vi "Measure Statistics (Multiple).vi"(6 "Measurements":T2[](array[typedef]), 8 "error in (no error)":errorcluster, 9 "No. Reads":i32, 10 "Channel":T3, 11 "MSOX6004 in":refnum<class "MSOX6004.lvclass">) -> (0 "error out":errorcluster, 2 "Multiple Statistics":T1(array[cluster]), 3 "MSOX6004 out":refnum<class "MSOX6004.lvclass">)   [LabVIEW 2018, in "MSOX6004.lvlib" / "MSOX6004.lvclass"]
uses:
  MSOX6004.lvclass
  PPLs/Oscilloscope/Parent/Oscilloscope.lvlibp/Custom Controls/Analog Channels.ctl
  PPLs/Oscilloscope/Parent/Oscilloscope.lvlibp/Custom Controls/Measurement.ctl
  MSOX6004.lvclass/MSOX6004.ctl
  <instrlib>/Keysight InfiniiVision/Keysight InfiniiVision.lvlib
  PPLs/Oscilloscope/Parent/Oscilloscope.lvlibp
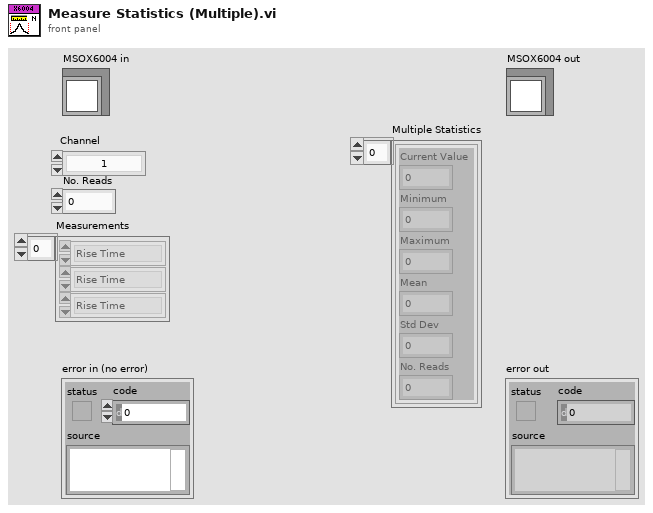
[diagram p1: front panel]
types:
  T1 = cluster{"Current Value":dbl, "Minimum":dbl, "Maximum":dbl, "Mean":dbl, "Std Dev":dbl, "No. Reads":dbl}[]
  T2 = typedef "Oscilloscope.lvlibp/Measurement.ctl" = enum16{"Rise Time", "Fall Time", "Frequency", "Period", "RMS (V)", "Peak-Peak (V)", "Max (V)", "Min (V)", "High State (V)", "Low State (V)", "Average (V)", "Width (Negative)", "Width (Positive)", "Duty Cycle (Negative)", "Duty Cycle (Positive)", "Amplitude", "Cycle RMS (V)", "Cycle Avg (V)", "Overshoot", "Preshoot", "Time at Max", "Frequency Counter", "Time at Min", "Delay", "Value at Time", "Phase", "Time at Value", "Time of Edge", "Area", "Burst Width", "Falling Edge Count", "Rising Edge Count", "Falling Pulse Count", "Rising Pulse Count", "Std Dev", "Pulse Width"}
  T3 = typedef "Oscilloscope.lvlibp/Analog Channels.ctl" = enum16{"1", "2", "3", "4", "5", "6", "7", "8", "9", "10", "11", "12", "13", "14", "15", "16"}
  T4 = cluster{"Current Value":dbl, "Minimum":dbl, "Maximum":dbl, "Mean":dbl, "Std Dev":dbl, "No. Reads":dbl}
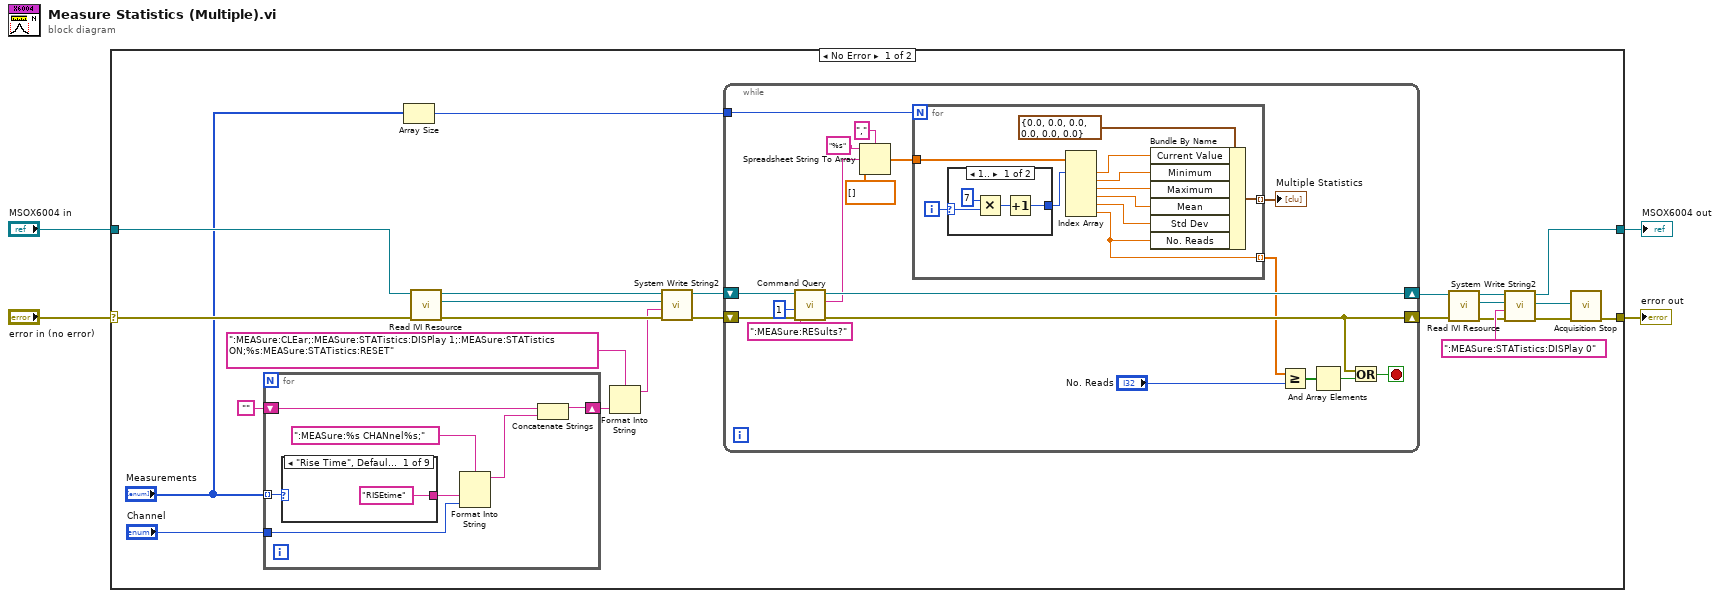
[diagram p0: block diagram]
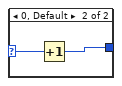
[diagram p2: hidden frame]
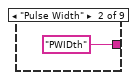
[diagram p3: hidden frame]
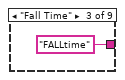
[diagram p4: hidden frame]
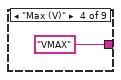
[diagram p5: hidden frame]
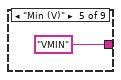
[diagram p6: hidden frame]
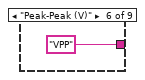
[diagram p7: hidden frame]
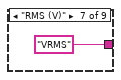
[diagram p8: hidden frame]
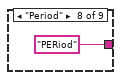
[diagram p9: hidden frame]
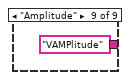
[diagram p10: hidden frame]
diagram:
  n1 = case shown="No Error" "error in (no error)" {
    selector: "error in (no error)" -> [w20 w78]
    tunnel: "MSOX6004 in" -> [w21 w79]
    tunnel: [w8 w79] -> w2
    tunnel: [w7 w78] -> w1
    frame No Error {
      n2 = for {
        tunnel: "Measurements" -> [w68] mode=indexing
        tunnel: "Channel" -> [w66]
        shift-right: [w64] -> w23
        shift-left: "" -> [w63]
        n3 = case shown="\"Rise Time\", Default" w68 {
          tunnel: ["RISEtime" "PWIDth" "FALLtime" "VMAX" "VMIN" "VPP" "VRMS" "PERiod" "VAMPlitude"] -> w67
          frame "Rise Time", Default {
          }
          frame "Pulse Width" {
          }
          frame "Fall Time" {
          }
          frame "Max (V)" {
          }
          frame "Min (V)" {
          }
          frame "Peak-Peak (V)" {
          }
          frame "RMS (V)" {
          }
          frame "Period" {
          }
          frame "Amplitude" {
          }
        }
        n4 = Format Into String(format string=":MEASure:%s CHANnel%s;", w67, w66) -> (resulting string=w62:string)  [unwired: 2 in, 1 out]
        n5 = Concatenate Strings(w63, w62) -> (w64:string)
      }
      n6 = Array Size(array="Measurements") -> (size(s)=w5:i32)
      n7 = call "Read IVI Resource.vi"("error in (no error)"=w20, "MSOX6004 in"=w21) -> ("error out"=w19:errorcluster, "IVI Resource"=w22:refnum<k15>, "MSOX6004 out"=w16:refnum<class "MSOX6004.lvclass">)  [unwired: 7 in]
      n8 = Format Into String(format string=":MEASure:CLEar;:MEASure:STATistics:DISPlay 1;:MEASure:STATistics ON;%s:MEASure:STATistics:RESET", w23) -> (resulting string=w18:string)  [unwired: 2 in, 1 out]
      n9 = call <instrlib>:"System Write String2.vi"("error in (no error)"=w19, "Data"=w18, "instrument handle"=w22) -> ("error out"=w17:errorcluster)  [unwired: 7 in, 1 out]
      n10 = while {
        shift-right: [w42] -> w9
        shift-left: w16 -> [w44]
        shift-right: [w36] -> w10
        shift-left: w17 -> [w43]
        tunnel: w5 -> [w33]
        stop <- w27 stop-if-true
        n11 = call "Command Query.vi"("error in (no error)"=w43, "Delay (ms)"=u32 1, "Command"=":MEASure:RESults?", "MSOX6004 in"=w44) -> ("error out"=w36:errorcluster, "Response"=w32:string, "MSOX6004 out"=w42:refnum<class "MSOX6004.lvclass">)  [unwired: 5 in]
        n12 = Spreadsheet String To Array(delimiter (Tab)=",", format string="%s", spreadsheet string=w32, array type (2D Dbl)=dbl[] []) -> (array=w40:dbl[])
        n13 = for {
          N: w33 -> [_]
          tunnel: w40 -> [w55]
          tunnel: [w46] -> w30 mode=indexing
          tunnel: [w45] -> w31 mode=indexing
          i -> [w54]
          n14 = case shown="1.." w54 {
            selector: w54 -> [w59 w61]
            tunnel: [w56 w60] -> w53
            frame 1.. {
              n15 = Multiply(x=7, y=w59) -> (x*y=w57:i32)
              n16 = Increment(x=w57) -> (x+1=w56:i32)
            }
            frame 0, Default {
              n17 = Increment(x=w61) -> (x+1=w60:i32)
            }
          }
          n18 = Index Array(array=w55, index #1=w53) -> (element #1=w51:dbl, element #2=w50:dbl, element #3=w49:dbl, element #4=w48:dbl, element #5=w47:dbl, element #6=w46:dbl)  [unwired: 5 in]
          n19 = Bundle By Name(cluster=T4 {"Current Value"=0.0, "Minimum"=0.0, "Maximum"=0.0, "Mean"=0.0, "Std Dev"=0.0, "No. Reads"=0.0} ("Statistics"), "Current Value"=w51, "Minimum"=w50, "Maximum"=w49, "Mean"=w48, "Std Dev"=w47, "No. Reads"=w46) -> (w45:T4)
        }
        "Multiple Statistics" <- w31
        n20 = Greater Or Equal?(x=w30, y="No. Reads") -> (x >= y?=w29:bool[])
        n21 = And Array Elements(Boolean array=w29) -> (logical AND=w28:bool)
        n22 = Or(x=w36, y=w28) -> (x .or. y?=w27:bool)
      }
      n23 = call "Read IVI Resource.vi"("error in (no error)"=w10, "MSOX6004 in"=w9) -> ("error out"=w12:errorcluster, "IVI Resource"=w15:refnum<k15>, "MSOX6004 out"=w8:refnum<class "MSOX6004.lvclass">)  [unwired: 7 in]
      n24 = call <instrlib>:"System Write String2.vi"("error in (no error)"=w12, "Data"=":MEASure:STATistics:DISPlay 0", "instrument handle"=w15) -> ("error out"=w11:errorcluster, "instrument handle out"=w13:refnum<k15>)  [unwired: 7 in]
      n25 = call <instrlib>:"Acquisition Stop.vi"("error in (no error)"=w11, "instrument handle"=w13) -> ("error out"=w7:errorcluster)  [unwired: 8 in, 1 out]
    }
    frame Error {
    }
  }
  "error out" <- w1
  "MSOX6004 out" <- w2
